vi "CSM_Tool_Launcher.vi"(6 "Variant in":variant, 7 "Shift Pressed?":bool, 8 "error in (no error)":errorcluster, 10 "QD Combo Box Ref":refnum<vi>, 11 "QD Launch VI Ref":refnum<vi>) -> (0 "error out":errorcluster, 4 "Variant out":variant)   [LabVIEW 2017]
doc: "Launches JKISM++ Tools Launcher.\n\nDefault Shortcut - [J]"
uses:
  user.lib/_NEVSTOP/Communicable State Machine(CSM)/_Shared/CSM Shared.lvlib
panel:
  out "appended path":path
  in  "Undo Name":string="Quick Drop Keyboard Shortcut"
  # "Do not change the connector pane of this VI.\n\nSee the block diagram for directions on how to use this template."
  # "Specify the name of the Undo transaction"
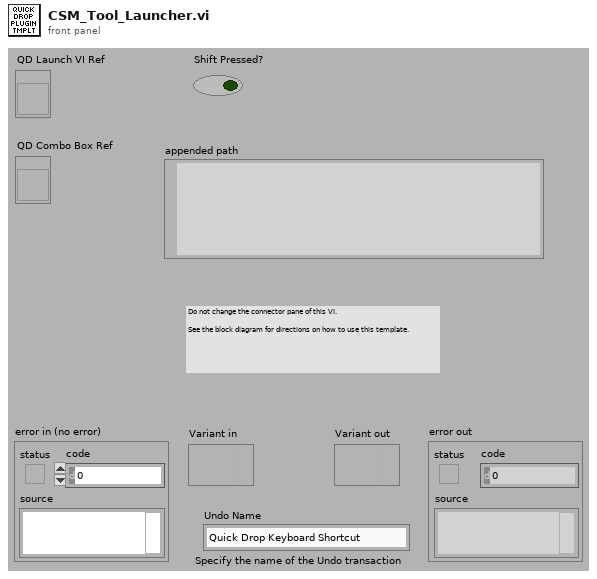
[diagram p1: front panel]
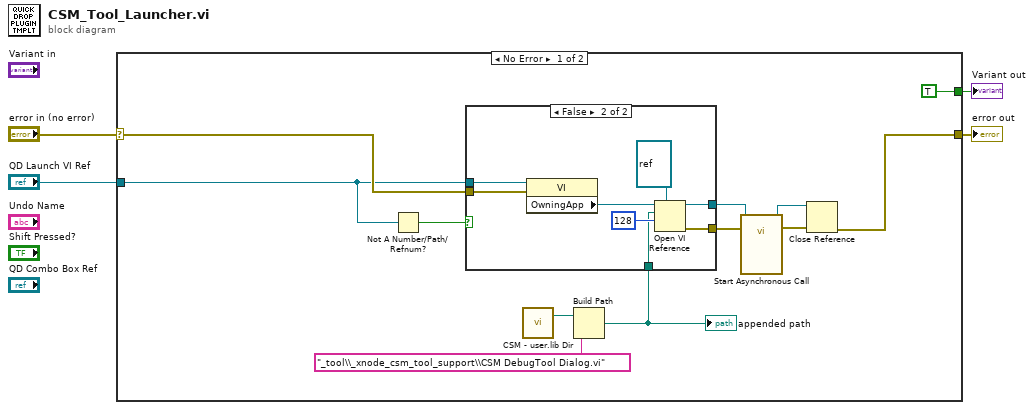
[diagram p0: block diagram]
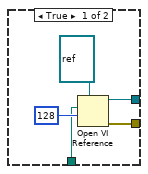
[diagram p2: hidden frame]
diagram:
  n1 = case shown="No Error" "error in (no error)" {
    selector: "error in (no error)" -> [w8 w30]
    tunnel: [w7 w30] -> w3
    tunnel: "QD Launch VI Ref" -> [w6 _]
    tunnel: [TRUE _] -> w1
    frame No Error {
      n2 = Not A Number/Path/Refnum?(number/path/refnum=w6) -> (NaN/Path/Refnum?=w5:bool)
      n3 = call "CSM - user.lib Dir.vi"() -> ("csm_user.lib_dir"=w9:path)  [unwired: 2 in, 1 out]
      n4 = Build Path(base path=w9, name or relative path="_tool\\_xnode_csm_tool_support\\CSM DebugTool Dialog.vi") -> (appended path=w10:path)
      "appended path" <- w10
      n5 = case shown="False" w5 {
        tunnel: [w20 w28] -> w12
        tunnel: [w19 w27] -> w11
        tunnel: w10 -> [w18 w26]
        tunnel: w8 -> [_ w24]
        tunnel: w6 -> [_ w23]
        frame True {
          n6 = Open VI Reference(type specifier VI Refnum (for type only)=refnum<vi> refnum, vi path=w18, options=128) -> (vi reference=w20:refnum<vi>, error out=w19:errorcluster)  [unwired: 3 in]
        }
        frame False {
          n7 = property class="VI"(reference=w23, error in=w24) -> ("OwningApp"=w22:refnum<vi>)  [unwired: 2 out]
          n8 = Open VI Reference(type specifier VI Refnum (for type only)=refnum<vi> refnum, application reference (local)=w22, vi path=w26, options=128) -> (vi reference=w28:refnum<vi>, error out=w27:errorcluster)  [unwired: 2 in]
        }
      }
      n9 = call-by-ref "Start Asynchronous Call"(reference=w12, error in=w11) -> (reference out=w14:refnum<vi>, error out=w13:errorcluster)  [unwired: 12 in]
      n10 = Close Reference(reference=w14, error in (no error)=w13) -> (error out=w7:errorcluster)
    }
    frame Error {
    }
  }
  "error out" <- w3
  "Variant out" <- w1
